vi "tb_interpolate accuracy.vi"() -> ()   [LabVIEW 2011]
uses:
  <vilib>/ptbypt/NI_PtbyPt.lvlib
  Controls/Interpolation Input Data.ctl
  Controls/ResampleVectorInfo (Single Point).ctl
  Controls/ResampleVectorInfo (Multiple Point).ctl
panel:
  in  "Resample Info":T1={"x[n].ResampleInfo"={"Calc Resample?"=TRUE, "Lambda"=0.5}, "x[n-1].ResampleInfo"={"Calc Resample?"=TRUE, "Lambda"=0.5}}
  out "Input Valid":bool[](array[boolean])
  out "Input X1":dbl[](array[numeric]) format="%.2f"
  out "Input X0":dbl[](array[numeric]) format="%.2f"
  out "Y1":T4(array[cluster])
  out "Y0":T4(array[cluster])
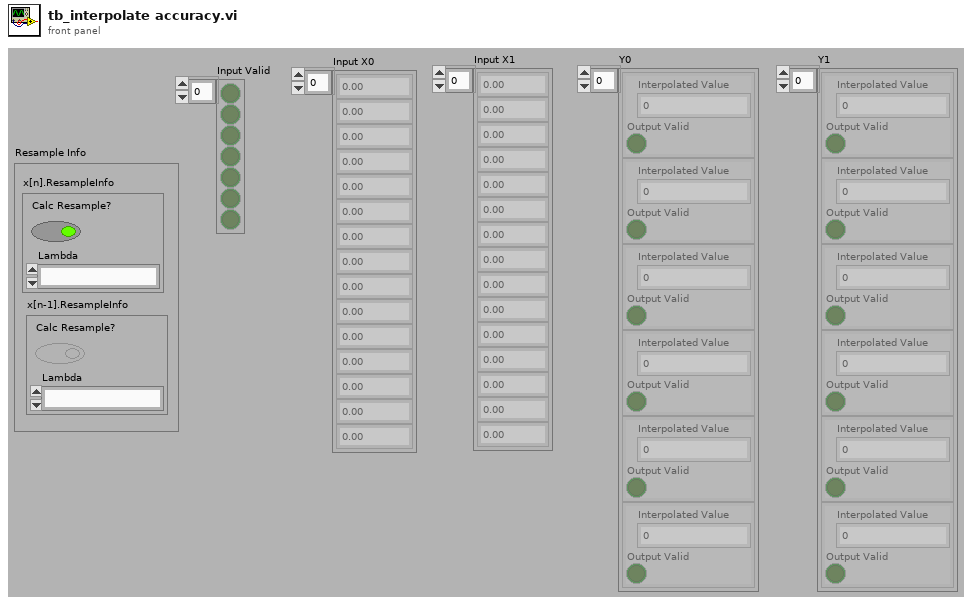
[diagram p1: front panel]
types:
  T1 = typedef "ResampleVectorInfo (Multiple Point).ctl" = cluster{"x[n].ResampleInfo":T2, "x[n-1].ResampleInfo":T2}
  T2 = typedef "ResampleVectorInfo (Single Point).ctl" = cluster{"Calc Resample?":bool, "Lambda":fxp<+/-,18,1>}
  T3 = typedef "Interpolation Input Data.ctl" = fxp<+/-,18,1>
  T4 = cluster{"Interpolated Value":T3, "Output Valid":bool}[]
  T5 = typedef "Interpolation Output Data.ctl" = fxp<+/-,19,1>
  T6 = cluster{"Interpolated Value":T5, "Output Valid":bool}
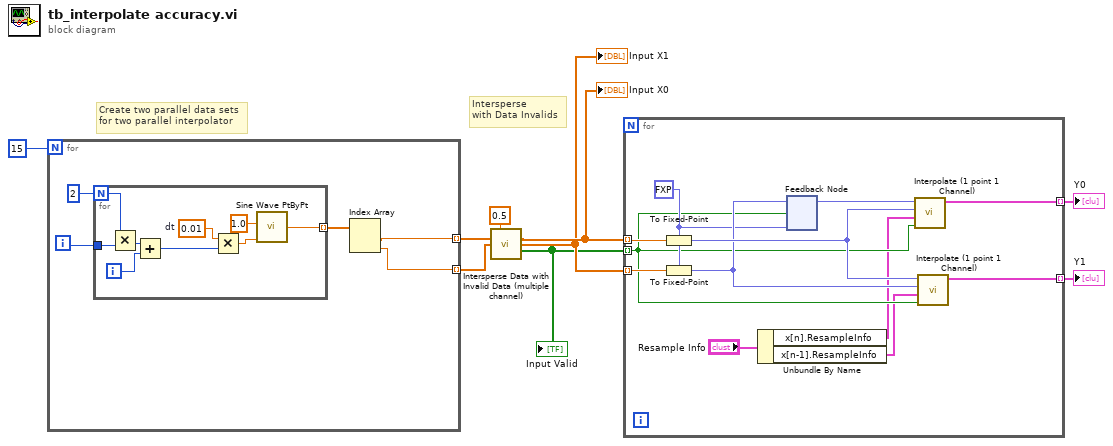
[diagram p0: block diagram]
diagram:
  # "Intersperse\nwith Data Invalids"
  # "Create two parallel data sets\nfor two parallel interpolator"
  n1 = for {
    N: 15 -> [_]
    tunnel: [w11] -> w6 mode=indexing
    tunnel: [w10] -> w5 mode=indexing
    i -> [w13]
    n2 = for {
      N: 2 -> [w18]
      tunnel: [w20] -> w14 mode=indexing
      tunnel: w13 -> [w19]
      i -> [w16]
      w22 = 0.01  # dt
      n3 = Multiply(x=w18, y=w19) -> (x*y=w17:i32)
      n4 = Add(x=w17, y=w16) -> (x+y=w15:i32)
      n5 = Multiply(x=w22, y=w15) -> (x*y=w21:dbl)
      n6 = call <vilib>:"Sine Wave PtByPt.vi"("time"=w21, "frequency"=1.0) -> ("sine wave"=w20:dbl)  [unwired: 2 in]
    }
    n7 = Index Array(array=w14) -> (element #1=w11:dbl, element #2=w10:dbl)  [unwired: 2 in]
  }
  n8 = call <userlib>:"Intersperse Data with Invalid Data (multiple channel).vi"("Intersperse Ratio"=0.5, "Channel0 Input"=w6, "Channel1 Input"=w5) -> ("Channel0 Output"=w4:dbl[], "Channel1 Output"=w3:dbl[], "Data Valid"=w2:bool[])  [unwired: 10 in]
  "Input X0" <- w4
  "Input X1" <- w3
  "Input Valid" <- w2
  n9 = for {
    tunnel: [w34] -> w8 mode=indexing
    tunnel: [w33] -> w7 mode=indexing
    tunnel: w3 -> [w30] mode=indexing
    tunnel: w4 -> [w32] mode=indexing
    tunnel: w2 -> [w27] mode=indexing
    w28 = fxp<+/-,16,1> 0.0
    n10 = To Fixed-Point(fixed-point type=w28, number=w32) -> (fixed-point=w31:fxp<+/-,16,1>)
    n11 = To Fixed-Point(fixed-point type=w28, number=w30) -> (fixed-point=w29:fxp<+/-,16,1>)
    n12 = Unbundle By Name("Resample Info") -> ("x[n].ResampleInfo"=w25:T2, "x[n-1].ResampleInfo"=w24:T2)
    n13 = feedback #1(w28) -> (w35:fxp<+/-,16,1>)
    n14 = feedback-in #1(w29, w27) -> ()
    n15 = call "Interpolate (1 point 1 Channel).vi"("Data Valid"=w27, "x[n].ResampleInfo"=w25, "Current Point.Value"=w31, "Previous Point.Value"=w35) -> ("Output Data"=w34:T6)  [unwired: 7 in]
    n16 = call "Interpolate (1 point 1 Channel).vi"("Data Valid"=w27, "x[n].ResampleInfo"=w24, "Current Point.Value"=w29, "Previous Point.Value"=w31) -> ("Output Data"=w33:T6)  [unwired: 7 in]
  }
  "Y0" <- w8
  "Y1" <- w7
